vi "WBRT Filter.vi"(8 "error in (no error)":errorcluster, 11 "WBRT State In":T1={"Encoders"={"Roll"=0.0, "Pitch"=0.0, "Yaw"=0.0, "Roll Trim"=0.0, "Pitch Trim"=0.0, "Yaw Trim"=0.0, "Roll Rate"=0.0, "Pitch Rate"=0.0, "Yaw Rate"=0.0}, "SPI Data"={"X-Gyro"=0.0, "Y-Gyro"=0.0, "Z-Gyro"=0.0, "X-Accel"=0.0, "Y-Accel"=0.0, "Z-Accel"=0.0}, "Camera"={"Numeric"=0.0}, "Filter Data"={"Filter Enabled?"=FALSE, "Filter Type"=enum."Equi-Ripple", "Pass Frequency"=1.0, "Stop Frequency (Equi-Ripple)"=0.45000000000000007, "Order"=0, "Ripple (dB)"=2.0}, "FPGA VI Reference"=refnum, "dt"=0.0, "Elapsed Time (msec)"=0, "Setpoints"={"Roll Setpoint (degrees)"=125.0, "Pitch Setpoint (degrees)"=125.0, "Yaw Setpoint (degrees)"=125.0}, "Commands"={"Left Command"=0.0, "Right Command"=0.0}, "Trajectory Data"=[], "Gains"={"Gain1"=0.0, "Gain2"=0.0, "Gain3"=0.0, "Gain4"=0.0, "Gain5"=0.0, "Gain6"=0.0, "Gain7"=0.0, "Gain8"=0.0, "Gain9"=0.0}, "Global Variables"={"Variable1"=[], "Variable2"=[], "Variable3"=[], "Variable4"=[]}, "Centroid"={"X Centroid"=0.0, "Y Centroid"=0.0}, "Error1"=0.0, "Error2"=0.0, "Error3"=0.0, "Error4"=0.0, "Recorded Data"=[], "Landing Factor"=0.0} {"Trajectory Data" format="%0.3f"; "Filter Data"."Stop Frequency (Equi-Ripple)" format="%0.3f"; "Filter Data"."Pass Frequency" format="%0.3f"}) -> (0 "error out":errorcluster, 3 "WBRT State Out":T1={"Encoders"={"Roll"=0.0, "Pitch"=0.0, "Yaw"=0.0, "Roll Trim"=0.0, "Pitch Trim"=0.0, "Yaw Trim"=0.0, "Roll Rate"=0.0, "Pitch Rate"=0.0, "Yaw Rate"=0.0}, "SPI Data"={"X-Gyro"=0.0, "Y-Gyro"=0.0, "Z-Gyro"=0.0, "X-Accel"=0.0, "Y-Accel"=0.0, "Z-Accel"=0.0}, "Camera"={"Numeric"=0.0}, "Filter Data"={"Filter Enabled?"=FALSE, "Filter Type"=enum."Equi-Ripple", "Pass Frequency"=1.0, "Stop Frequency (Equi-Ripple)"=0.45000000000000007, "Order"=0, "Ripple (dB)"=2.0}, "FPGA VI Reference"=refnum, "dt"=0.0, "Elapsed Time (msec)"=0, "Setpoints"={"Roll Setpoint (degrees)"=125.0, "Pitch Setpoint (degrees)"=125.0, "Yaw Setpoint (degrees)"=125.0}, "Commands"={"Left Command"=0.0, "Right Command"=0.0}, "Trajectory Data"=[], "Gains"={"Gain1"=0.0, "Gain2"=0.0, "Gain3"=0.0, "Gain4"=0.0, "Gain5"=0.0, "Gain6"=0.0, "Gain7"=0.0, "Gain8"=0.0, "Gain9"=0.0}, "Global Variables"={"Variable1"=[], "Variable2"=[], "Variable3"=[], "Variable4"=[]}, "Centroid"={"X Centroid"=0.0, "Y Centroid"=0.0}, "Error1"=0.0, "Error2"=0.0, "Error3"=0.0, "Error4"=0.0, "Recorded Data"=[], "Landing Factor"=0.0} {"Trajectory Data" format="%0.3f"; "Filter Data"."Stop Frequency (Equi-Ripple)" format="%0.3f"; "Filter Data"."Pass Frequency" format="%0.3f"})   [LabVIEW 2012]
doc: "Filters the acquired encoder data. There are three filter available:\n\nEqui-Ripple (FIR)\nButtorworth (IIR)\nChebyshev (IIR)\n\nAll three encoders go through the same filter configuration.\n\nAuthor: Brandon Steele\n\nCopyright: Brigham Young University"
uses:
  Custom Controls/WBRT State.ctl
  Custom Controls/WBRT Encoders.ctl
  Custom Controls/WBRT SPI Data.ctl
  Custom Controls/WBRT Filter Data.ctl
  Custom Controls/WBRT Filter Type.ctl
  FPGA Samples/spi_single port_example/Host API/Controls/FPGA SPI_FPGA Ref.ctl
  Custom Controls/WBRT Setpoints.ctl
  Custom Controls/WBRT Commands.ctl
  Custom Controls/WBRT Gains.ctl
  Custom Controls/WBRT Global Variables.ctl
  <vilib>/Analysis/3filter.llb/Filter Passband Type.ctl
  <vilib>/ptbypt/NI_PtbyPt.lvlib
  <vilib>/Analysis/NI_AALBase.lvlib
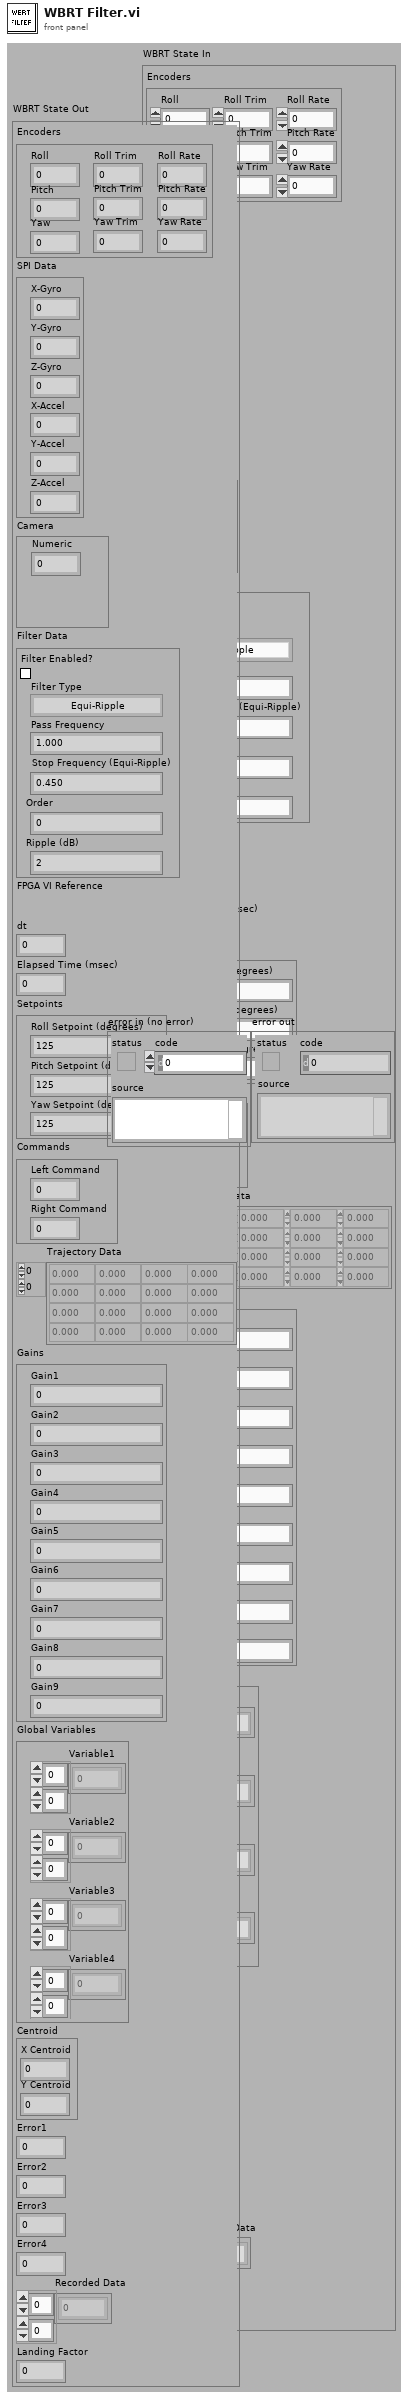
[diagram p1: front panel]
types:
  T1 = typedef "WBRT State.ctl" = cluster{"Encoders":T2, "SPI Data":T3, "Camera":cluster{"Numeric":dbl}, "Filter Data":T4, "FPGA VI Reference":T6, "dt":dbl, "Elapsed Time (msec)":u32, "Setpoints":T7, "Commands":T8, "Trajectory Data":dbl[][], "Gains":T9, "Global Variables":T10, "Centroid":cluster{"X Centroid":sgl, "Y Centroid":sgl}, "Error1":dbl, "Error2":dbl, "Error3":dbl, "Error4":dbl, "Recorded Data":dbl[][], "Landing Factor":dbl}
  T2 = typedef "WBRT Encoders.ctl" = cluster{"Roll":dbl, "Pitch":dbl, "Yaw":dbl, "Roll Trim":dbl, "Pitch Trim":dbl, "Yaw Trim":dbl, "Roll Rate":dbl, "Pitch Rate":dbl, "Yaw Rate":dbl}
  T3 = typedef "WBRT SPI Data.ctl" = cluster{"X-Gyro":dbl, "Y-Gyro":dbl, "Z-Gyro":dbl, "X-Accel":dbl, "Y-Accel":dbl, "Z-Accel":dbl}
  T4 = typedef "WBRT Filter Data.ctl" = cluster{"Filter Enabled?":bool, "Filter Type":T5, "Pass Frequency":dbl, "Stop Frequency (Equi-Ripple)":dbl, "Order":i32, "Ripple (dB)":dbl}
  T5 = typedef "WBRT Filter Type.ctl" = enum16{"Equi-Ripple", "Butterworth", "Chebyshev"}
  T6 = typedef "FPGA SPI_FPGA Ref.ctl" = refnum<k20>
  T7 = typedef "WBRT Setpoints.ctl" = cluster{"Roll Setpoint (degrees)":dbl, "Pitch Setpoint (degrees)":dbl, "Yaw Setpoint (degrees)":dbl}
  T8 = typedef "WBRT Commands.ctl" = cluster{"Left Command":dbl, "Right Command":dbl}
  T9 = typedef "WBRT Gains.ctl" = cluster{"Gain1":dbl, "Gain2":dbl, "Gain3":dbl, "Gain4":dbl, "Gain5":dbl, "Gain6":dbl, "Gain7":dbl, "Gain8":dbl, "Gain9":dbl}
  T10 = typedef "WBRT Global Variables.ctl" = cluster{"Variable1":dbl[][], "Variable2":dbl[][], "Variable3":dbl[][], "Variable4":dbl[][]}
  T11 = typedef "NI_AALBase.lvlib/Filter Passband Type.ctl" = enum32{"Lowpass", "Highpass", "Bandpass", "Bandstop"}
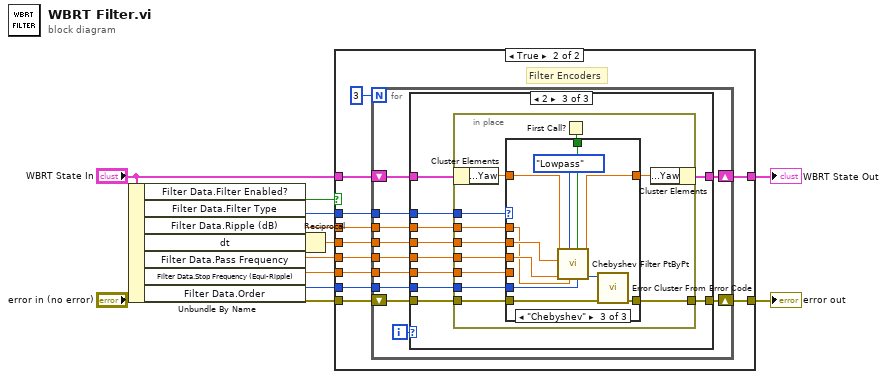
[diagram p0: block diagram]
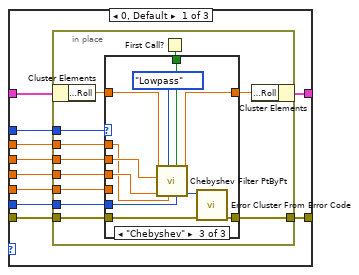
[diagram p3: hidden frame]
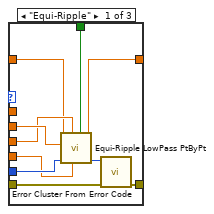
[diagram p4: hidden frame]
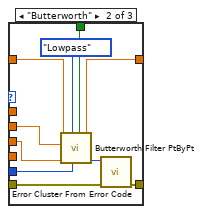
[diagram p5: hidden frame]
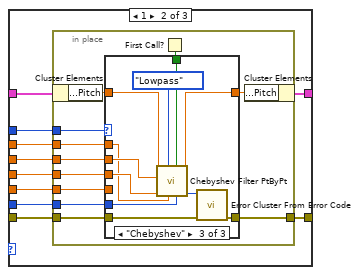
[diagram p6: hidden frame]
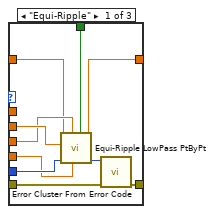
[diagram p7: hidden frame]
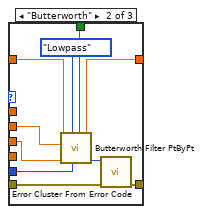
[diagram p8: hidden frame]
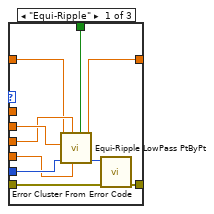
[diagram p9: hidden frame]
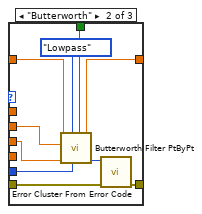
[diagram p10: hidden frame]
diagram:
  n1 = Unbundle By Name("WBRT State In") -> ("Filter Data.Filter Enabled?"=w12:bool, "Filter Data.Filter Type"=w7:T5, "Filter Data.Ripple (dB)"=w2:dbl, "dt"=w6:dbl, "Filter Data.Pass Frequency"=w5:dbl, "Filter Data.Stop Frequency (Equi-Ripple)"=w4:dbl, "Filter Data.Order"=w3:i32)
  n2 = Reciprocal(x=w6) -> (1/x=w1:dbl)
  n3 = case shown="True" w12 {
    tunnel: "WBRT State In" -> [w14 w16]
    tunnel: [w14 w15] -> w10
    tunnel: "error in (no error)" -> [w13 w25]
    tunnel: [w13 w24] -> w8
    tunnel: w7 -> [_ w23]
    tunnel: w1 -> [_ w22]
    tunnel: w5 -> [_ w21]
    tunnel: w4 -> [_ w20]
    tunnel: w3 -> [_ w19]
    tunnel: w2 -> [_ w18]
    frame False {
    }
    frame True {
      # "Filter Encoders"
      n4 = for {
        N: 3 -> [_]
        tunnel: w23 -> [w34]
        tunnel: w22 -> [w33]
        tunnel: w21 -> [w32]
        tunnel: w20 -> [w31]
        tunnel: w19 -> [w30]
        tunnel: w18 -> [w29]
        shift-right: [w35] -> w24
        shift-left: w25 -> [w36]
        shift-right: [w26] -> w15
        shift-left: w16 -> [w27]
        i -> [w28]
        n5 = case shown="2" w28 {
          tunnel: w36 -> [w46 w98 w150]
          tunnel: [w45 w97 w149] -> w35
          tunnel: w34 -> [w44 w96 w148]
          tunnel: w33 -> [w43 w95 w147]
          tunnel: w32 -> [w42 w94 w146]
          tunnel: w31 -> [w41 w93 w145]
          tunnel: w30 -> [w40 w92 w144]
          tunnel: w29 -> [w39 w91 w143]
          tunnel: w27 -> [w38 w90 w142]
          tunnel: [w37 w89 w141] -> w26
          frame 0, Default {
            n6 = in-place {
              in-place-border: w46 -> [w57]
              in-place-border: [w56] -> w45
              in-place-border: w44 -> [w55]
              in-place-border: w43 -> [w54]
              in-place-border: w42 -> [w53]
              in-place-border: w41 -> [w52]
              in-place-border: w40 -> [w51]
              in-place-border: w39 -> [w49]
              n7 = in-place-cluster #1(w38) -> ("Encoders.Roll"=w48:dbl)
              n8 = First Call?() -> (First Call?: T/F=w50:bool)
              n9 = case shown="\"Chebyshev\"" w55 {
                tunnel: w57 -> [w66 w76 w87]
                tunnel: [w65 w75 w86] -> w56
                tunnel: w54 -> [w62 w72 w83]
                tunnel: w53 -> [w61 w71 w82]
                tunnel: w52 -> [w63 _ _]
                tunnel: w51 -> [w64 w70 w81]
                tunnel: w50 -> [w60 w73 w84]
                tunnel: w49 -> [_ _ w80]
                tunnel: w48 -> [w59 w69 w79]
                tunnel: [w58 w68 w78] -> w47
                frame "Equi-Ripple" {
                  n10 = call <vilib>:"Equi-Ripple LowPass PtByPt.vi"("initialize"=w60, "stop freq"=w63, "pass freq"=w61, "# of taps"=w64, "sampling freq: fs"=w62, "x"=w59) -> ("error"=w67:i32, "Filtered x"=w58:dbl)  [unwired: 3 in]
                  n11 = call <vilib>:"Error Cluster From Error Code.vi"("error in (no error)"=w66, "error code (0)"=w67) -> ("error out"=w65:errorcluster)  [unwired: 7 in]
                }
                frame "Butterworth" {
                  n12 = call <vilib>:"Butterworth Filter PtByPt.vi"("initialize"=w73, "order"=w70, "filter type"=Filter_Passband_Type."Lowpass", "low cutoff freq: fl"=w71, "sampling freq: fs"=w72, "x"=w69) -> ("error"=w77:i32, "Filtered x"=w68:dbl)  [unwired: 3 in]
                  n13 = call <vilib>:"Error Cluster From Error Code.vi"("error in (no error)"=w76, "error code (0)"=w77) -> ("error out"=w75:errorcluster)  [unwired: 7 in]
                }
                frame "Chebyshev" {
                  n14 = call <vilib>:"Chebyshev Filter PtByPt.vi"("order"=w81, "initialize"=w84, "ripple(dB)"=w80, "filter type"=Filter_Passband_Type."Lowpass", "low cutoff freq: fl"=w82, "sampling freq: fs"=w83, "x"=w79) -> ("error"=w88:i32, "Filtered x"=w78:dbl)  [unwired: 3 in]
                  n15 = call <vilib>:"Error Cluster From Error Code.vi"("error in (no error)"=w87, "error code (0)"=w88) -> ("error out"=w86:errorcluster)  [unwired: 7 in]
                }
              }
              n16 = in-place-cluster #1("Encoders.Roll"=w47) -> (w37:T1)
            }
          }
          frame 1 {
            n17 = in-place {
              in-place-border: w98 -> [w109]
              in-place-border: [w108] -> w97
              in-place-border: w96 -> [w107]
              in-place-border: w95 -> [w106]
              in-place-border: w94 -> [w105]
              in-place-border: w93 -> [w104]
              in-place-border: w92 -> [w103]
              in-place-border: w91 -> [w101]
              n18 = in-place-cluster #2(w90) -> ("Encoders.Pitch"=w100:dbl)
              n19 = First Call?() -> (First Call?: T/F=w102:bool)
              n20 = case shown="\"Chebyshev\"" w107 {
                tunnel: w109 -> [w118 w128 w139]
                tunnel: [w117 w127 w138] -> w108
                tunnel: w106 -> [w114 w124 w135]
                tunnel: w105 -> [w113 w123 w134]
                tunnel: w104 -> [w115 _ _]
                tunnel: w103 -> [w116 w122 w133]
                tunnel: w102 -> [w112 w125 w136]
                tunnel: w101 -> [_ _ w132]
                tunnel: w100 -> [w111 w121 w131]
                tunnel: [w110 w120 w130] -> w99
                frame "Equi-Ripple" {
                  n21 = call <vilib>:"Equi-Ripple LowPass PtByPt.vi"("initialize"=w112, "stop freq"=w115, "pass freq"=w113, "# of taps"=w116, "sampling freq: fs"=w114, "x"=w111) -> ("error"=w119:i32, "Filtered x"=w110:dbl)  [unwired: 3 in]
                  n22 = call <vilib>:"Error Cluster From Error Code.vi"("error in (no error)"=w118, "error code (0)"=w119) -> ("error out"=w117:errorcluster)  [unwired: 7 in]
                }
                frame "Butterworth" {
                  n23 = call <vilib>:"Butterworth Filter PtByPt.vi"("initialize"=w125, "order"=w122, "filter type"=Filter_Passband_Type."Lowpass", "low cutoff freq: fl"=w123, "sampling freq: fs"=w124, "x"=w121) -> ("error"=w129:i32, "Filtered x"=w120:dbl)  [unwired: 3 in]
                  n24 = call <vilib>:"Error Cluster From Error Code.vi"("error in (no error)"=w128, "error code (0)"=w129) -> ("error out"=w127:errorcluster)  [unwired: 7 in]
                }
                frame "Chebyshev" {
                  n25 = call <vilib>:"Chebyshev Filter PtByPt.vi"("order"=w133, "initialize"=w136, "ripple(dB)"=w132, "filter type"=Filter_Passband_Type."Lowpass", "low cutoff freq: fl"=w134, "sampling freq: fs"=w135, "x"=w131) -> ("error"=w140:i32, "Filtered x"=w130:dbl)  [unwired: 3 in]
                  n26 = call <vilib>:"Error Cluster From Error Code.vi"("error in (no error)"=w139, "error code (0)"=w140) -> ("error out"=w138:errorcluster)  [unwired: 7 in]
                }
              }
              n27 = in-place-cluster #2("Encoders.Pitch"=w99) -> (w89:T1)
            }
          }
          frame 2 {
            n28 = in-place {
              in-place-border: w150 -> [w161]
              in-place-border: [w160] -> w149
              in-place-border: w148 -> [w159]
              in-place-border: w147 -> [w158]
              in-place-border: w146 -> [w157]
              in-place-border: w145 -> [w156]
              in-place-border: w144 -> [w155]
              in-place-border: w143 -> [w153]
              n29 = in-place-cluster #3(w142) -> ("Encoders.Yaw"=w152:dbl)
              n30 = First Call?() -> (First Call?: T/F=w154:bool)
              n31 = case shown="\"Chebyshev\"" w159 {
                tunnel: w161 -> [w170 w180 w191]
                tunnel: [w169 w179 w190] -> w160
                tunnel: w158 -> [w166 w176 w187]
                tunnel: w157 -> [w165 w175 w186]
                tunnel: w156 -> [w167 _ _]
                tunnel: w155 -> [w168 w174 w185]
                tunnel: w154 -> [w164 w177 w188]
                tunnel: w153 -> [_ _ w184]
                tunnel: w152 -> [w163 w173 w183]
                tunnel: [w162 w172 w182] -> w151
                frame "Equi-Ripple" {
                  n32 = call <vilib>:"Equi-Ripple LowPass PtByPt.vi"("initialize"=w164, "stop freq"=w167, "pass freq"=w165, "# of taps"=w168, "sampling freq: fs"=w166, "x"=w163) -> ("error"=w171:i32, "Filtered x"=w162:dbl)  [unwired: 3 in]
                  n33 = call <vilib>:"Error Cluster From Error Code.vi"("error in (no error)"=w170, "error code (0)"=w171) -> ("error out"=w169:errorcluster)  [unwired: 7 in]
                }
                frame "Butterworth" {
                  n34 = call <vilib>:"Butterworth Filter PtByPt.vi"("initialize"=w177, "order"=w174, "filter type"=Filter_Passband_Type."Lowpass", "low cutoff freq: fl"=w175, "sampling freq: fs"=w176, "x"=w173) -> ("error"=w181:i32, "Filtered x"=w172:dbl)  [unwired: 3 in]
                  n35 = call <vilib>:"Error Cluster From Error Code.vi"("error in (no error)"=w180, "error code (0)"=w181) -> ("error out"=w179:errorcluster)  [unwired: 7 in]
                }
                frame "Chebyshev" {
                  n36 = call <vilib>:"Chebyshev Filter PtByPt.vi"("order"=w185, "initialize"=w188, "ripple(dB)"=w184, "filter type"=Filter_Passband_Type."Lowpass", "low cutoff freq: fl"=w186, "sampling freq: fs"=w187, "x"=w183) -> ("error"=w192:i32, "Filtered x"=w182:dbl)  [unwired: 3 in]
                  n37 = call <vilib>:"Error Cluster From Error Code.vi"("error in (no error)"=w191, "error code (0)"=w192) -> ("error out"=w190:errorcluster)  [unwired: 7 in]
                }
              }
              n38 = in-place-cluster #3("Encoders.Yaw"=w151) -> (w141:T1)
            }
          }
        }
      }
    }
  }
  "WBRT State Out" <- w10
  "error out" <- w8
